vi "Do.vi"(8 "error in":errorcluster, 10 "Actor in":refnum<class "Actor.lvclass">, 11 "Change AutoCycle Params MSG":refnum<class "Change AutoCycle Params MSG.lvclass">) -> (0 "error out":errorcluster, 2 "Actor out":refnum<class "Actor.lvclass">)   [LabVIEW 2016, in "Change AutoCycle Params MSG.lvclass"]
doc: "(<B>Filename</B>: Actor Framework.lvlib:Message.lvclass:Do.vi)\n\nDefines what a message does when it is received by an actor. Generally, a message instructs an actor to invoke one of its methods. By default, this method does nothing. A child class must override it to define behavior. Create a child class by using the Actor Framework Message Maker dialog box."
uses:
  Change AutoCycle Params MSG.lvclass
  <vilib>/ActorFramework/Actor/Actor.lvclass
  Change AutoCycle Params MSG.lvclass/Change AutoCycle Params MSG.ctl
  gController.lvclass
  C:/Program Files (x86)/National Instruments/LabVIEW 2016/vi.lib/MSR Consulting, LLC/General Reuse/SuperActor/SuperActor.lvclass
  C:/Program Files (x86)/National Instruments/LabVIEW 2016/vi.lib/ActorFramework/Actor/Actor.lvclass
  <vilib>/MSR Consulting, LLC/General Reuse/SuperActor/SuperActor.lvclass/SuperActor.ctl
  <vilib>/MSR Consulting, LLC/General Reuse/SuperActor/Read Log Session.vi
  <vilib>/MSR Consulting, LLC/General Reuse/SuperActor/Read CVT Session.vi
  <vilib>/MSR Consulting, LLC/General Reuse/Session APIs/_Session Fwk/Session - Root.lvclass
  <vilib>/MSR Consulting, LLC/General Reuse/Session APIs/CVT/CVT.lvclass
  <vilib>/MSR Consulting, LLC/General Reuse/Session APIs/Session Log/System Log.lvclass
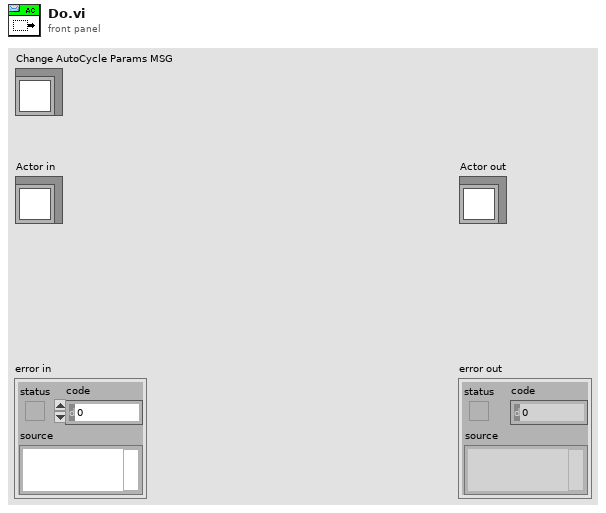
[diagram p1: front panel]
types:
  T1 = typedef "Session - Root.lvclass/Session Handle.ctl" = refnum<data-value>
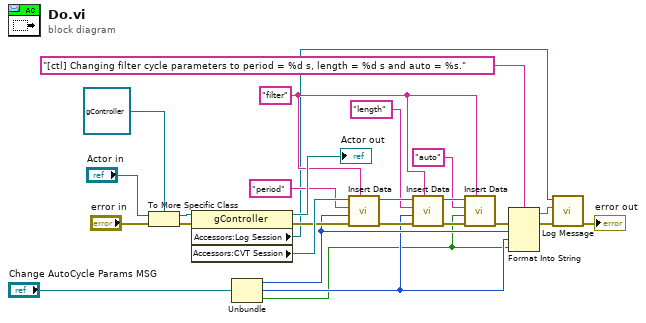
[diagram p0: block diagram]
diagram:
  w16 = "filter" ("Group")
  n1 = To More Specific Class(target class=refnum<class "gController.lvclass"> refnum ("Controller.lvlib:gController"), reference="Actor in", error in="error in") -> (specific class reference=w22:refnum<class "gController.lvclass">, error out=w9:errorcluster)
  n2 = property class="gController"(reference=w22, error in=w9) -> (reference out=→"Actor out":refnum<class "gController.lvclass">, error out=w13:errorcluster, "Accessors:Log Session"=w10:T1, "Accessors:CVT Session"=w20:T1)
  n3 = Unbundle("Change AutoCycle Params MSG") -> (w7:i32, w6:i32, w5:bool)
  n4 = call <vilib>:"Insert Data.vi"("Group"=w16, "error in"=w13, "Data"=w7, "tag"="period", "CVT Session In"=w20) -> ("error out"=w12:errorcluster, "CVT Session Out"=w18:T1)  [unwired: 5 in]
  n5 = call <vilib>:"Insert Data.vi"("Group"=w16, "error in"=w12, "Data"=w6, "tag"="length", "CVT Session In"=w18) -> ("error out"=w11:errorcluster, "CVT Session Out"=w15:T1)  [unwired: 5 in]
  n6 = call <vilib>:"Insert Data.vi"("Group"=w16, "error in"=w11, "Data"=w5, "tag"="auto", "CVT Session In"=w15) -> ("error out"=w4:errorcluster)  [unwired: 5 in, 1 out]
  n7 = Format Into String(format string="[ctl] Changing filter cycle parameters to period = %d s, length = %d s and auto = %s.", error in=w4, w7, w6, w5) -> (resulting string=w2:string, error out=w3:errorcluster)  [unwired: 1 in]
  n8 = call <vilib>:"Log Message.vi"("error in"=w3, "MSG In"=w2, "session in"=w10) -> ("error out"=→"error out":errorcluster)  [unwired: 7 in, 1 out]
